vi "get_stream_dimensions.vi"(3 "error in":errorcluster, 5 "Sensor configuration":string) -> (0 "error out":errorcluster, 1 "y":i32, 2 "x":i32)   [LabVIEW 2019]
doc: "Get the dimensions from the camera configuration."
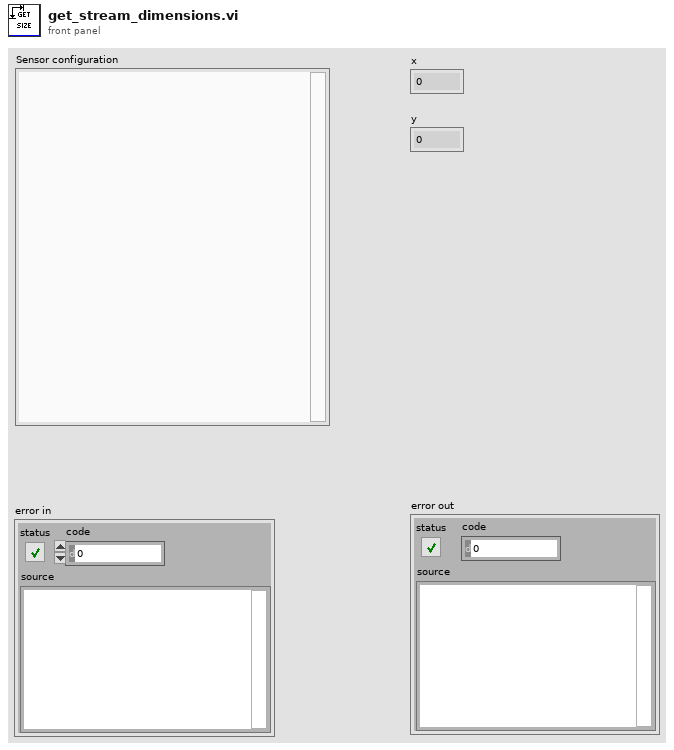
[diagram p1: front panel]
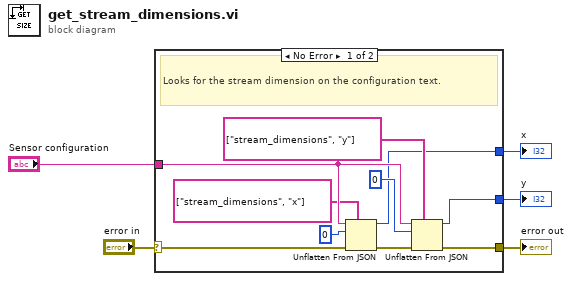
[diagram p0: block diagram]
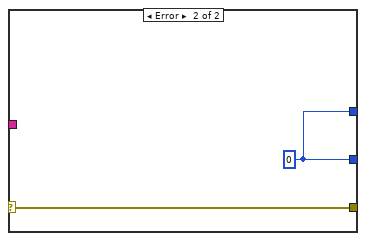
[diagram p2: hidden frame]
diagram:
  n1 = case shown="No Error" "error in" {
    selector: "error in" -> [w11 w16]
    tunnel: "Sensor configuration" -> [w13 _]
    tunnel: [w6 w17] -> w3
    tunnel: [w7 w17] -> w2
    tunnel: [w10 w16] -> w1
    frame No Error {
      # "Looks for the stream dimension on the configuration text."
      n2 = Unflatten From JSON(path=string[] ["stream_dimensions", "x"], JSON string=w13, type and defaults=0 ("x dimension"), error in (no error)=w11) -> (value=w7:i32, error out=w12:errorcluster)  [unwired: 3 in]
      n3 = Unflatten From JSON(path=string[] ["stream_dimensions", "y"], JSON string=w13, type and defaults=0 ("x dimension"), error in (no error)=w12) -> (value=w6:i32, error out=w10:errorcluster)  [unwired: 3 in]
    }
    frame Error {
      w17 = 0
    }
  }
  "y" <- w3
  "x" <- w2
  "error out" <- w1
